vi "SendProcessedData.vi"(5 "Median":dbl, 7 "Mean":dbl, 8 "error in (no error)":errorcluster, 9 "RMS":dbl, 10 "Duration":dbl) -> (0 "error out":errorcluster)   [LabVIEW 2019, in "SignalProcessor.lvlib"]
doc: "This event broadcasts processed data from audio signal\n_____\nCreated using Delacor QMH Event Scripter 4.2.1.88."
uses:
  SignalProcessor.lvlib
  SendProcessedData Argument--cluster.ctl
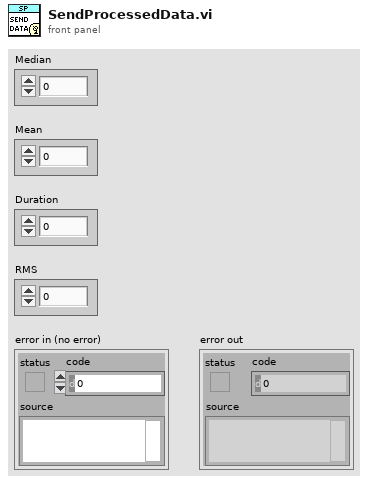
[diagram p1: front panel]
types:
  T1 = typedef "SignalProcessor.lvlib/SendProcessedData Argument--cluster.ctl" = cluster{"Duration":dbl, "RMS":dbl, "Mean":dbl, "Median":dbl}
  T2 = typedef "SignalProcessor.lvlib/Broadcast Events--cluster.ctl" = cluster{"Module Did Init":refnum<user-event>, "Status Updated":refnum<user-event>, "Error Reported":refnum<user-event>, "Module Did Stop":refnum<user-event>, "Update Module Execution Status":refnum<user-event>, "SendProcessedData":refnum<user-event>}
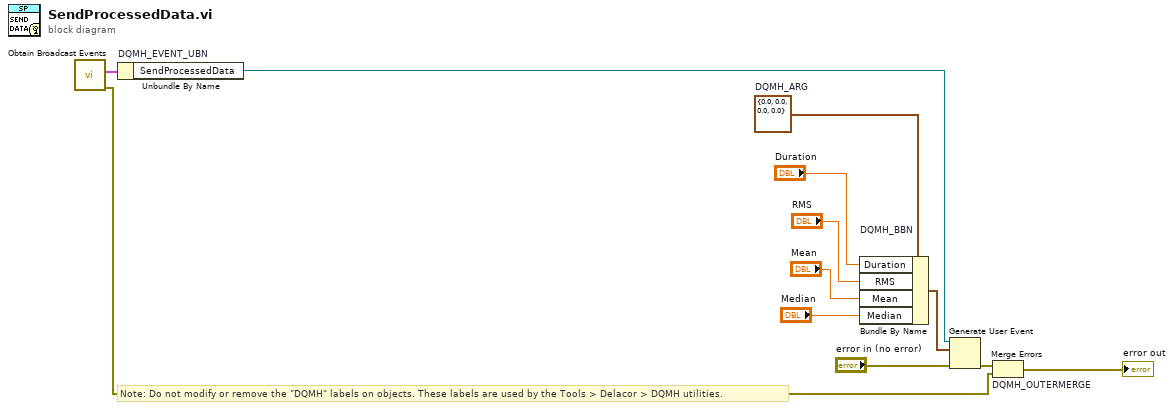
[diagram p0: block diagram]
diagram:
  w7 = T1 {"Duration"=0.0, "RMS"=0.0, "Mean"=0.0, "Median"=0.0}  # DQMH_ARG
  # "Note: Do not modify or remove the \"DQMH\" labels on objects. These labels are used by the Tools > Delacor > DQMH utilities."
  n1 = call "Obtain Broadcast Events.vi"() -> ("error out"=w2:errorcluster, "SignalProcessor Broadcast Events"=w1:T2)  [unwired: 10 in]
  n2 = Unbundle By Name "DQMH_EVENT_UBN"(w1) -> ("SendProcessedData"=w9:refnum<user-event>)
  n3 = Bundle By Name "DQMH_BBN"(cluster=w7, "Duration"="Duration", "RMS"="RMS", "Mean"="Mean", "Median"="Median") -> (w10:T1)
  n4 = Generate User Event(user event=w9, event data cluster=w10, error in="error in (no error)") -> (error out=w8:errorcluster)  [unwired: 1 in, 1 out]
  n5 = Merge Errors "DQMH_OUTERMERGE"(w8, w2) -> (→"error out":errorcluster)
